vi "Initialization VI.vi"(8 "error in (no error)":errorcluster, 10 "Custom XML":string, 11 "Device Item Ref in":T1 format="%.0x") -> (0 "error out":errorcluster, 3 "Device Item Ref out":T1 format="%.0x")   [LabVIEW 2021, in "DSF System Explorer.lvlib"]
uses:
  DSF System Explorer.lvlib
  Shared/DSF Shared.lvlib
  Includes/DSF Core.lvlibp/Typedefs/DSF FIFO Options.ctl
  Includes/DSF Core.lvlibp/Classes/Thread/Thread Options.ctl
  Includes/DSF Core.lvlibp/Typedefs/DSF Plugin Options.ctl
  Includes/DSF Core.lvlibp/Typedefs/DSF Performance Options.ctl
  Includes/DSF Core.lvlibp/Classes/Framework/Data Server Options.ctl
  Includes/DSF Core.lvlibp/Classes/Framework/Framework Options.ctl
  <vilib>/NI VeriStand/Custom Device API/Custom Device Item Ref.ctl
  <vilib>/NI VeriStand/Custom Device API/Custom Device API.lvlib
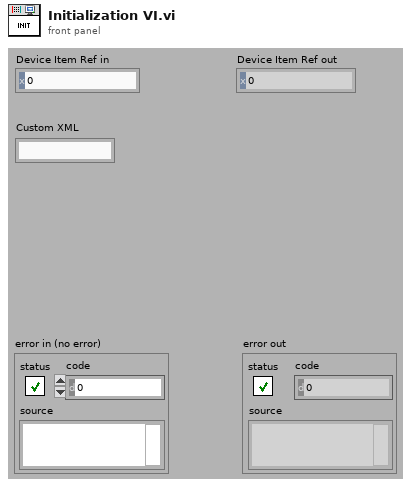
[diagram p1: front panel]
types:
  T1 = typedef "Custom Device API.lvlib/Custom Device Item Ref.ctl" = u64
  T2 = typedef "DSF Core.lvlibp/Framework.lvclass/Framework Options.ctl" = cluster{"FIFO Options":T3, "Thread Options":T4, "Plugin Options":T5, "Performance Options":T6, "Data Server Options":T7}
  T3 = typedef "DSF Core.lvlibp/Framework.lvclass/DSF FIFO Options.ctl" = cluster{"Infinite Timeouts":bool}
  T4 = typedef "DSF Core.lvlibp/Thread.lvclass/Thread Options.ctl" = cluster{"Show FP On Call":bool, "Close FP After Call":bool, "Allow Debugging":bool}
  T5 = typedef "DSF Core.lvlibp/Framework.lvclass/DSF Plugin Options.ctl" = cluster{"Default Components":bool}
  T6 = typedef "DSF Core.lvlibp/DSF Performance Options.ctl" = cluster{"Measure Period":bool, "Measure Rx/Tx Duration":bool}
  T7 = typedef "DSF Core.lvlibp/Framework.lvclass/Data Server Options.ctl" = cluster{"Enable Data Server":bool, "Period":u32}
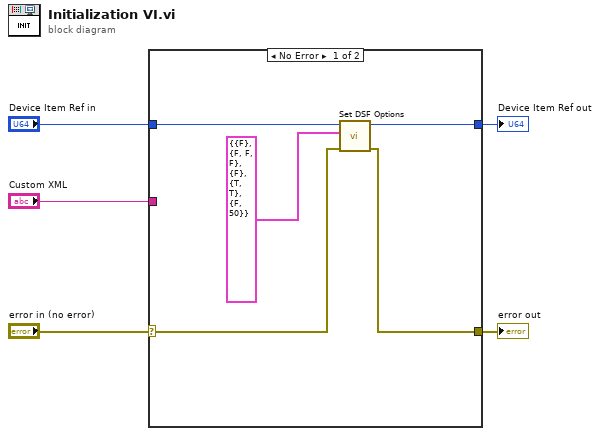
[diagram p0: block diagram]
diagram:
  n1 = case shown="No Error" "error in (no error)" {
    selector: "error in (no error)" -> [w9 w12]
    tunnel: [w6 w12] -> w5
    tunnel: [w7 w11] -> w3
    tunnel: "Device Item Ref in" -> [w10 w11]
    tunnel: "Custom XML" -> [_ _]
    frame No Error {
      n2 = call "Set DSF Options.vi"("error in (no error)"=w9, "options"=T2 {"FIFO Options"={"Infinite Timeouts"=FALSE}, "Thread Options"={"Show FP On Call"=FALSE, "Close FP After Call"=FALSE, "Allow Debugging"=FALSE}, "Plugin Options"={"Default Components"=FALSE}, "Performance Options"={"Measure Period"=TRUE, "Measure Rx/Tx Duration"=TRUE}, "Data Server Options"={"Enable Data Server"=FALSE, "Period"=50}}, "Item Ref in"=w10) -> ("error out"=w6:errorcluster, "Item Ref out"=w7:T1)  [unwired: 7 in]
    }
    frame Error {
    }
  }
  "error out" <- w5
  "Device Item Ref out" <- w3
